vi "extract plot data.vi"(8 "data in":T1) -> (0 "data out":T1, 3 "plotData":dbl[](array[numeric]))   [LabVIEW 2018]
uses:
  liveData cluster.ctl
  type defs/liveArray.ctl
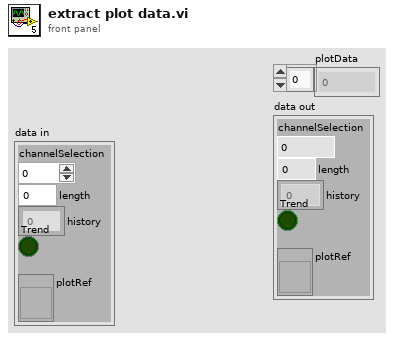
[diagram p1: front panel]
types:
  T1 = typedef "liveData cluster.ctl" = cluster{"channelSelection":i32, "length":dbl, "history":dbl[], "Trend":bool, "plotRef":refnum<vi>}
  T2 = typedef "localSharedVariables.lvlib/liveArray.ctl" = cluster{"ID":u32, "data":dbl[][], "updateRate":u32}
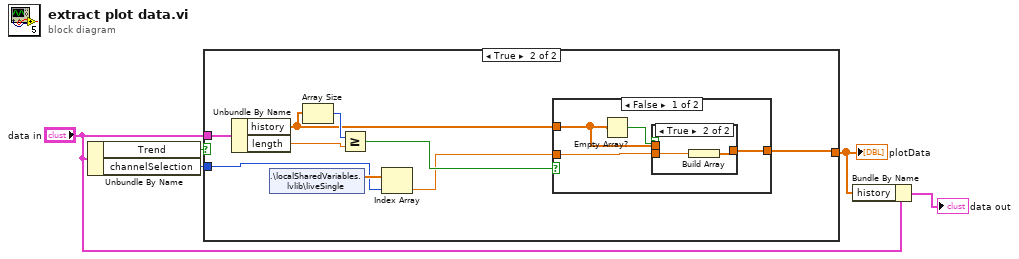
[diagram p0: block diagram]
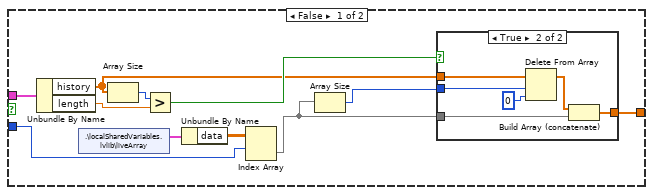
[diagram p2: hidden frame]
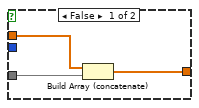
[diagram p3: hidden frame]
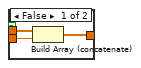
[diagram p4: hidden frame]
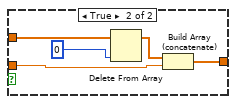
[diagram p5: hidden frame]
diagram:
  n1 = Unbundle By Name("data in") -> ("Trend"=w4:bool, "channelSelection"=w5:i32)
  n2 = case shown="True" w4 {
    tunnel: w5 -> [w14 w26]
    tunnel: "data in" -> [w9 w29]
    tunnel: [w8 w27] -> w2
    frame False {
      n3 = Unbundle By Name(w9) -> ("history"=w11:dbl[], "length"=w13:dbl)
      n4 = shared-variable ".\\localSharedVariables.lvlib\\liveArray"() -> (w16:T2)  [unwired: 1 in, 1 out]
      n5 = Array Size(array=w11) -> (size(s)=w10:i32)
      n6 = Greater?(x=w10, y=w13) -> (0:w12:bool)
      n7 = Unbundle By Name(w16) -> ("data"=w15:dbl[][])
      n8 = Index Array(array=w15, index (row)=w14) -> (element=w7:dbl[])  [unwired: 1 in]
      n9 = Array Size(array=w7) -> (size(s)=w6:i32)
      n10 = case shown="True" w12 {
        tunnel: w7 -> [w18 w21]
        tunnel: w11 -> [w19 w23]
        tunnel: [w17 w20] -> w8
        tunnel: w6 -> [_ w25]
        frame False {
          n11 = Build Array (concatenate)(w19, w18) -> (w17:dbl[])
        }
        frame True {
          n12 = Delete From Array(array=w23, length=w25, index=0) -> (array with subset deleted=w22:dbl[])  [unwired: 1 out]
          n13 = Build Array (concatenate)(w22, w21) -> (w20:dbl[])
        }
      }
    }
    frame True {
      n14 = Unbundle By Name(w29) -> ("history"=w32:dbl[], "length"=w30:dbl)
      n15 = shared-variable ".\\localSharedVariables.lvlib\\liveSingle"() -> (w34:dbl[])  [unwired: 1 in, 1 out]
      n16 = Array Size(array=w32) -> (size(s)=w33:i32)
      n17 = Greater Or Equal?(x=w33, y=w30) -> (x >= y?=w31:bool)
      n18 = Index Array(array=w34, index=w26) -> (element=w28:dbl)
      n19 = case shown="False" w31 {
        tunnel: w32 -> [w36 w47]
        tunnel: [w38 w45] -> w27
        tunnel: w28 -> [w37 w44]
        frame False {
          n20 = Empty Array?(array=w36) -> (empty?=w35:bool)
          n21 = case shown="True" w35 {
            tunnel: [w41 w42] -> w38
            tunnel: w37 -> [w40 w43]
            tunnel: w36 -> [w39 _]
            frame False {
              n22 = Build Array (concatenate)(w39, w40) -> (w41:dbl[])
            }
            frame True {
              n23 = Build Array(w43) -> (w42:dbl[])
            }
          }
        }
        frame True {
          n24 = Delete From Array(array=w47, index=0) -> (array with subset deleted=w46:dbl[])  [unwired: 1 in, 1 out]
          n25 = Build Array (concatenate)(w46, w44) -> (w45:dbl[])
        }
      }
    }
  }
  "plotData" <- w2
  n26 = Bundle By Name(cluster="data in", "history"=w2) -> (→"data out":T1)
